vi "Write Spectrum Configuration.vi"(8 "error in (no error)":errorcluster, 10 "Configuration":T1={"Start frequency"=500000.0, "End frequency"=2000000.0, "Coarse step"=40.0, "Step duration"=0.004, "Red Pitaya address"="192.168.1.100", "Open plot \non start"=FALSE, "Regions width"=0.0, "Fine step"=1.0, "Pause between scans"=0.0, "Clear rgs on start"=FALSE, "Output amplitude"=1.0} {"Output amplitude" min=0.0 max=1.0 step=0.1 format="%#_6pV"; "Pause between scans" format="%#_6ps"; "Fine step" min=0.001 format="%#_6pHz"; "Regions width" format="%#_6pHz"; "Step duration" format="%#_6ps"; "Coarse step" format="%#_6pHz"; "End frequency" format="%#_6pHz"; "Start frequency" format="%#_6pHz"}, 11 "Red Pitaya Transceiver Driver in":refnum<class "Red Pitaya Transceiver Driver.lvclass">) -> (0 "error out":errorcluster, 3 "Red Pitaya Transceiver Driver out":refnum<class "Red Pitaya Transceiver Driver.lvclass">)   [LabVIEW 2016, in "Red Pitaya Transceiver Driver.lvclass"]
uses:
  Red Pitaya Transceiver Driver.lvclass
  C:/github/NHMFL_Core/Libraries/Instruments/Instrument Driver/Instrument Driver.lvclass
  Spectrum Configuration.ctl
  Instruments/Instrument Driver/Write User configuration.vi
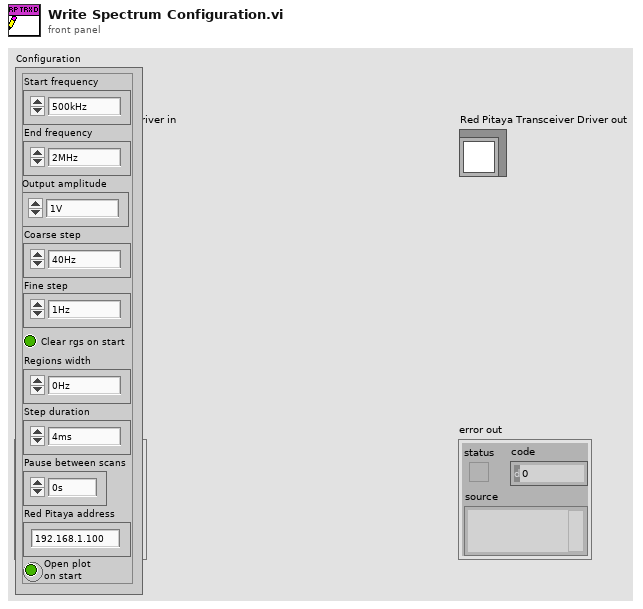
[diagram p1: front panel]
types:
  T1 = typedef "Spectrum Configuration.ctl" = cluster{"Start frequency":dbl, "End frequency":dbl, "Coarse step":dbl, "Step duration":dbl, "Red Pitaya address":string, "Open plot \non start":bool, "Regions width":dbl, "Fine step":dbl, "Pause between scans":dbl, "Clear rgs on start":bool, "Output amplitude":dbl}
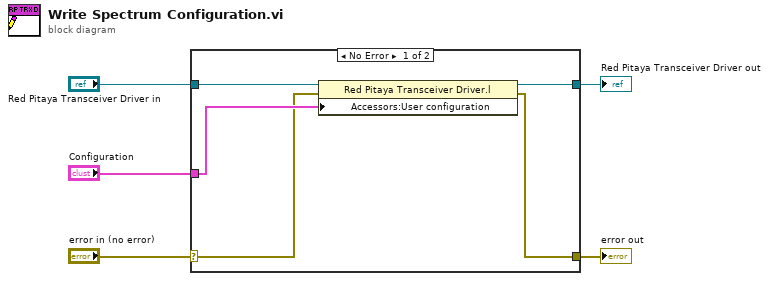
[diagram p0: block diagram]
diagram:
  n1 = case shown="No Error" "error in (no error)" {
    selector: "error in (no error)" -> [w7 w11]
    tunnel: [w6 w11] -> w4
    tunnel: [w9 w12] -> w2
    tunnel: "Red Pitaya Transceiver Driver in" -> [w10 w12]
    tunnel: "Configuration" -> [w8 _]
    frame No Error {
      n2 = property class="Red Pitaya Transceiver Driver.l"(reference=w10, error in=w7, "Accessors:User configuration"=w8) -> (reference out=w9:refnum<class "Red Pitaya Transceiver Driver.lvclass">, error out=w6:errorcluster)
    }
    frame Error {
    }
  }
  "error out" <- w4
  "Red Pitaya Transceiver Driver out" <- w2
